vi "LstDevGetId.vi"(7 "error in (no error)":errorcluster, 9 "dwId in":u32) -> (0 "error out":errorcluster, 1 "dwProductId":u32, 2 "dwId out":u32)   [LabVIEW 2018, in "LibTiePie.lvlib"]
uses:
  LibTiePie.lvlib
  LabViewHS4/libtiepie.dll
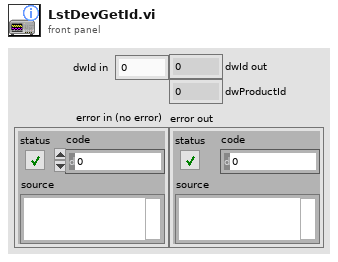
[diagram p1: front panel]
types:
  T1 = enum32{"Reserved1", "Product ID", "Index", "Reserved3", "Serial"}
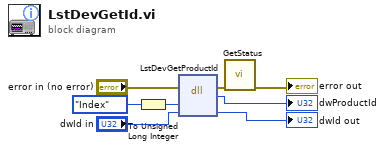
[diagram p0: block diagram]
diagram:
  n1 = To Unsigned Long Integer(number=T1."Index" ("Indentifier")) -> (unsigned 32bit integer=w6:u32)
  n2 = dll-call lib="C:/Users/cwaha/Documents/LabViewHS4/libtiepie.dll" fn="LstDevGetProductId"(error in="error in (no error)", "dwIdKind"=w6, "dwProductId"="dwId in") -> (error out=w3:errorcluster, "return type"=→"dwProductId":u32, "dwProductId"=→"dwId out":u32)  [unwired: 3 in, 1 out]
  n3 = call "GetStatus.vi"("error in (no error)"=w3) -> ("error out"=→"error out":errorcluster)  [unwired: 10 in]
